vi "Tosca-Initialize Visual Display.vi"(0 "Picture in":refnum<vi>, 5 "This VI":refnum<vi>, 7 "Visual Display Settings":T1) -> (8 "Array":cdb[][](array[numeric]), 10 "photodiode mask":u8[][](array[numeric]), 15 "error out":errorcluster)   [LabVIEW 2020]
uses:
  Tosca-Visual Display Settings.ctl
  epl-vi-lib/Utility VIs/Math VIs/LinSpace (x0-dx-npts).vi
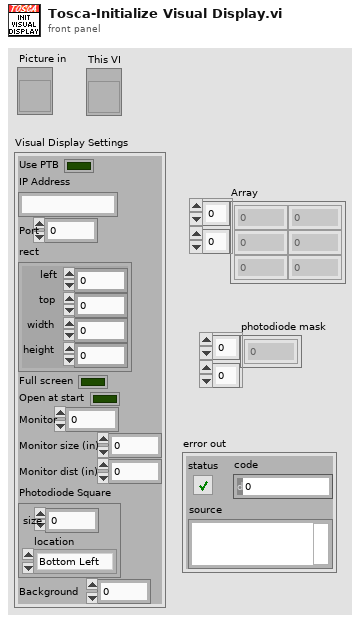
[diagram p1: front panel]
types:
  T1 = typedef "Tosca-Visual Display Settings.ctl" = cluster{"Use PTB":bool, "IP Address":string, "Port":i32, "rect":cluster{"left":i16, "top":i16, "width":i16, "height":i16}, "Full screen":bool, "Open at start":bool, "Monitor":i32, "Monitor size (in)":dbl, "Monitor dist (in)":dbl, "Photodiode Square":cluster{"size":i16, "location":enum16{"Bottom Left", "Top Left", "Top Right", "Bottom Right"}}, "Background":dbl}
  T2 = enum16{"Bottom Left", "Top Left", "Top Right", "Bottom Right"}
  T3 = cluster{"left":i16, "top":i16, "width":i16, "height":i16}
  T4 = typedef "LVAllMonitorsDisplayTypeDef.ctl" = cluster{"Bounds":cluster{"Left":i16, "Top":i16, "Right":i16, "Bottom":i16}, "Depth":i16}[]
  T5 = cluster{"Bounds":cluster{"Left":i16, "Top":i16, "Right":i16, "Bottom":i16}, "Depth":i16}
  T6 = cluster{"Left":i16, "Top":i16, "Right":i16, "Bottom":i16}
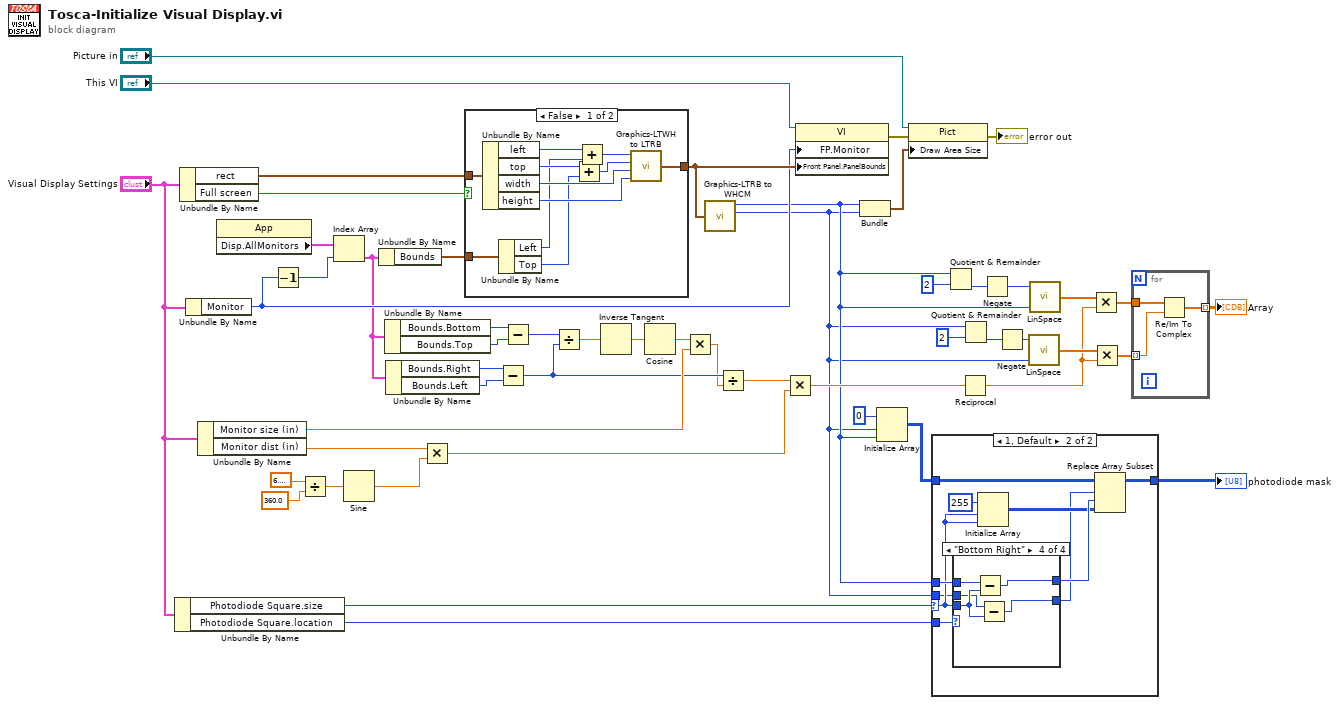
[diagram p0: block diagram]
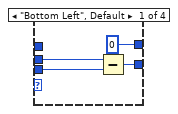
[diagram p3: hidden frame]
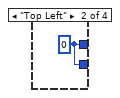
[diagram p4: hidden frame]
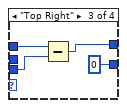
[diagram p5: hidden frame]
diagram:
  n1 = Unbundle By Name("Visual Display Settings") -> ("Photodiode Square.size"=w4:i16, "Photodiode Square.location"=w2:T2)
  n2 = Unbundle By Name("Visual Display Settings") -> ("rect"=w47:T3, "Full screen"=w48:bool)
  n3 = Unbundle By Name("Visual Display Settings") -> ("Monitor"=w42:i32)
  n4 = Unbundle By Name("Visual Display Settings") -> ("Monitor size (in)"=w31:dbl, "Monitor dist (in)"=w25:dbl)
  n5 = property class="App"() -> ("Disp.AllMonitors"=w44:T4)  [unwired: 2 in, 2 out]
  n6 = Decrement(x=w42) -> (x-1=w43:i32)
  n7 = Divide(x=6.283185307179586, y=360.0) -> (x/y=w26:dbl)
  n8 = Index Array(array=w44, index=w43) -> (element=w36:T5)
  n9 = Sine(x=w26) -> (sin(x)=w24:dbl)
  n10 = Unbundle By Name(w36) -> ("Bounds"=w41:T6)
  n11 = Unbundle By Name(w36) -> ("Bounds.Bottom"=w38:i16, "Bounds.Top"=w37:i16)
  n12 = Unbundle By Name(w36) -> ("Bounds.Right"=w40:i16, "Bounds.Left"=w39:i16)
  n13 = Multiply(x=w25, y=w24) -> (x*y=w22:dbl)
  n14 = case shown="False" w48 {
    tunnel: [w58 w64] -> w45
    tunnel: w47 -> [w59 _]
    tunnel: w41 -> [w57 w64]
    frame False {
      n15 = Unbundle By Name(w59) -> ("left"=w63:i16, "top"=w62:i16, "width"=w61:i16, "height"=w60:i16)
      n16 = Unbundle By Name(w57) -> ("Left"=w55:i16, "Top"=w53:i16)
      n17 = Add(x=w62, y=w53) -> (x+y=w54:i16)
      n18 = Add(x=w63, y=w55) -> (x+y=w56:i16)
      n19 = call "Graphics-LTWH to LTRB.vi"("Left"=w56, "Top"=w54, "Width"=w61, "Height"=w60) -> ("TLRB"=w58:T6)  [unwired: 4 in]
    }
    frame True {
    }
  }
  n20 = Subtract(x=w40, y=w39) -> (x-y=w30:i16)
  n21 = Subtract(x=w38, y=w37) -> (x-y=w35:i16)
  n22 = Divide(x=w35, y=w30) -> (x/y=w34:dbl)
  n23 = Inverse Tangent(1:w34) -> (0:w33:dbl)
  n24 = Cosine(x=w33) -> (cos(x)=w32:dbl)
  n25 = Multiply(x=w32, y=w31) -> (x*y=w29:dbl)
  n26 = call "Graphics-LTRB to WHCM.vi"("LTRB"=w45) -> ("Height"=w3:i16, "Width"=w5:i16)  [unwired: 4 in, 2 out]
  n27 = Divide(x=w30, y=w29) -> (x/y=w23:dbl)
  n28 = Multiply(x=w23, y=w22) -> (x*y=w21:dbl)
  n29 = property class="VI"(reference="This VI", "FP.Monitor"=w42, "Front Panel.PanelBounds"=w45) -> (error out=w52:errorcluster)  [unwired: 1 in, 1 out]
  n30 = Bundle("Width"=w5, "Height"=w3) -> (w51:cluster{"Width":i16, "Height":i16})  [unwired: 1 in]
  n31 = Initialize Array(u8 0, w3, w5) -> (w6:u8[][])
  n32 = property on="Property Node" class="Pict"(reference="Picture in", error in=w52, "Draw Area Size"=w51) -> (error out=→"error out":errorcluster)  [unwired: 1 out]
  n33 = case shown="1, Default" w4 {
    selector: w4 -> [_ w72]
    tunnel: w6 -> [w65 w74]
    tunnel: w5 -> [_ w73]
    tunnel: w3 -> [_ w71]
    tunnel: w2 -> [_ w70]
    tunnel: [w65 w66] -> w1
    frame 0 {
    }
    frame 1, Default {
      n34 = case shown="\"Bottom Right\"" w70 {
        tunnel: w73 -> [_ _ w83 w88]
        tunnel: w72 -> [w77 _ w81 w87]
        tunnel: w71 -> [w78 _ _ w85]
        tunnel: [0 w80 w82 w89] -> w69
        tunnel: [w76 w80 0 w86] -> w67
        frame "Bottom Left", Default {
          n35 = Subtract(x=w78, y=w77) -> (x-y=w76:i16)
        }
        frame "Top Left" {
          w80 = 0
        }
        frame "Top Right" {
          n36 = Subtract(x=w83, y=w81) -> (x-y=w82:i16)
        }
        frame "Bottom Right" {
          n37 = Subtract(x=w88, y=w87) -> (x-y=w89:i16)
          n38 = Subtract(x=w85, y=w87) -> (x-y=w86:i16)
        }
      }
      n39 = Initialize Array(u8 255, w72, w72) -> (w68:u8[][])
      n40 = Replace Array Subset(array=w74, new element=w68, index (row)=w67, index (col)=w69) -> (w66:u8[][])
    }
  }
  "photodiode mask" <- w1
  n41 = Quotient & Remainder(x=w5, y=i16 2) -> (floor(x/y)=w19:i16)  [unwired: 1 out]
  n42 = Reciprocal(x=w21) -> (1/x=w10:dbl)
  n43 = Quotient & Remainder(x=w3, y=i16 2) -> (floor(x/y)=w14:i16)  [unwired: 1 out]
  n44 = Negate(x=w19) -> (-x=w15:i16)
  n45 = Negate(x=w14) -> (-x=w13:i16)
  n46 = call-poly "LinSpace.vi"("npts"=w3, "x0"=w13) -> ("Array"=w11:dbl[])  [unwired: 2 in, 1 out]
  n47 = call-poly "LinSpace.vi"("npts"=w5, "x0"=w15) -> ("Array"=w18:dbl[])  [unwired: 2 in, 1 out]
  n48 = Multiply(x=w18, y=w10) -> (x*y=w17:dbl[])
  n49 = Multiply(x=w11, y=w10) -> (x*y=w9:dbl[])
  n50 = for {
    tunnel: w17 -> [w92]
    tunnel: [w90] -> w16 mode=indexing
    tunnel: w9 -> [w91] mode=indexing
    n51 = Re/Im To Complex(1:w91, 2:w92) -> (0:w90:cdb[])
  }
  "Array" <- w16
